vi "Write Numeric.vi"(8 "error in (no error)":errorcluster, 10 "Abs_Numeric.lvclass":refnum<class "Abs_Numeric.lvclass">, 11 "Reciprocal_Numeric in":refnum<class "Reciprocal_Numeric.lvclass">) -> (0 "error out":errorcluster, 3 "Reciprocal_Numeric out":refnum<class "Reciprocal_Numeric.lvclass">)   [LabVIEW 2021, in "Reciprocal_Numeric.lvclass"]
uses:
  Reciprocal_Numeric.lvclass
  Abs_Types/Numeric/Abs_Numeric.lvclass
  Reciprocal_Numeric.lvclass/Reciprocal_Numeric.ctl
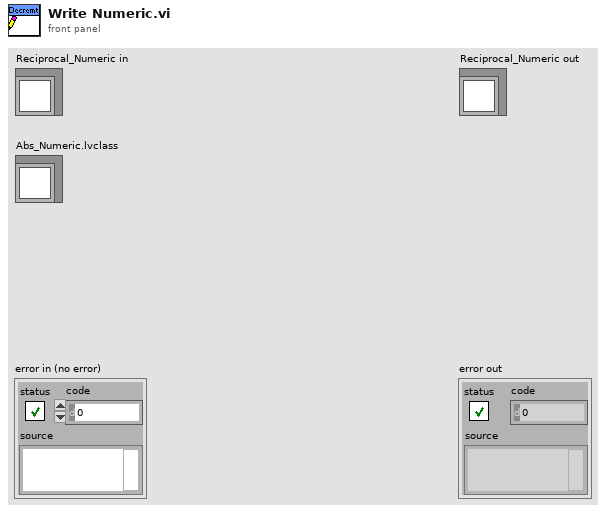
[diagram p1: front panel]
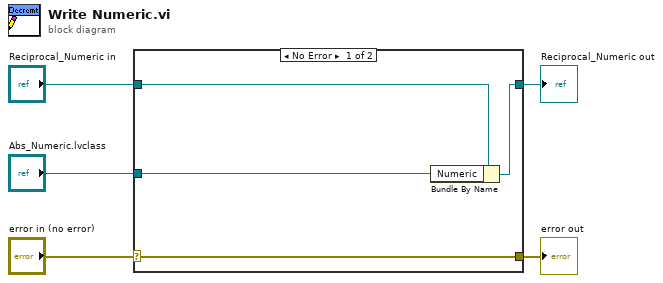
[diagram p0: block diagram]
diagram:
  n1 = case shown="No Error" "error in (no error)" {
    selector: "error in (no error)" -> [w9 w10]
    tunnel: [w9 w10] -> w4
    tunnel: [w7 w11] -> w2
    tunnel: "Reciprocal_Numeric in" -> [w8 w11]
    tunnel: "Abs_Numeric.lvclass" -> [w6 _]
    frame No Error {
      n2 = Bundle By Name(cluster=w8, "Numeric"=w6) -> (w7:refnum<class "Reciprocal_Numeric.lvclass">)
    }
    frame Error {
    }
  }
  "error out" <- w4
  "Reciprocal_Numeric out" <- w2
